vi "Rows Indexing with Feedback.vi"(9 "Boolean 2":bool, 10 "Boolean":bool, 11 "Array 3":i32[][](array[numeric])) -> (2 "Array":i32[](array[numeric]), 3 "Array 2":i32[](array[numeric]))   [LabVIEW 2014]
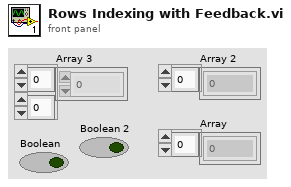
[diagram p1: front panel]
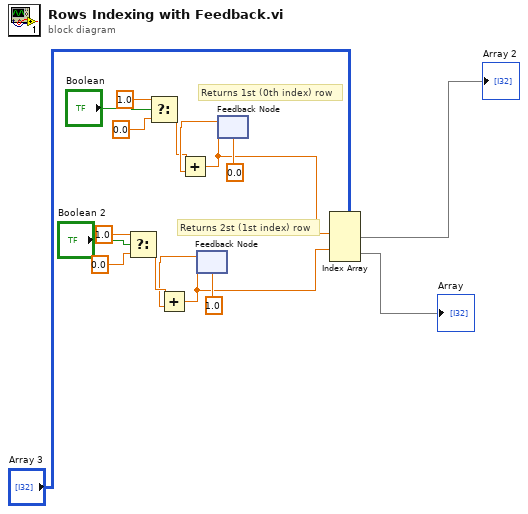
[diagram p0: block diagram]
diagram:
  # "Returns 2st (1st index) row"
  # "Returns 1st (0th index) row"
  n1 = Select(t=1.0, s="Boolean 2", f=0.0) -> (s? t:f=w13:dbl)
  n2 = Select(t=1.0, s="Boolean", f=0.0) -> (s? t:f=w7:dbl)
  n3 = feedback #1(1.0) -> (w11:dbl)
  n4 = Add(x=w13, y=w11) -> (x+y=w15:dbl)
  n5 = feedback-in #1(w15) -> ()
  n6 = feedback #2(0.0) -> (w10:dbl)
  n7 = Add(x=w7, y=w10) -> (x+y=w8:dbl)
  n8 = feedback-in #2(w8) -> ()
  n9 = Index Array(array="Array 3", index (row) #1=w8, index (row) #2=w15) -> (element #1=→"Array 2":i32[], element #2=→"Array":i32[])  [unwired: 2 in]
